vi "Wrap value.vi"(1 "Starting Angle":dbl min=0.0 max=360.0 step=1.0, 2 "Change":dbl) -> (0 "Num":dbl)   [LabVIEW 2016]
doc: "Essentially the mod function.....\n\nCreated by Team 4130 for use in the 2016-2017 FRC season"
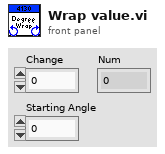
[diagram p1: front panel]
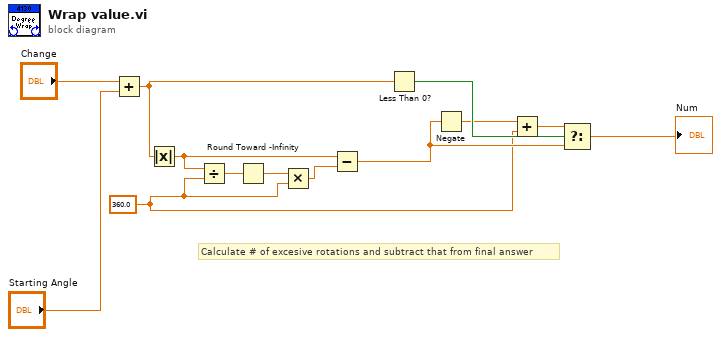
[diagram p0: block diagram]
diagram:
  w6 = 360.0
  # "Calculate # of excesive rotations and subtract that from final answer"
  n1 = Add(x="Change", y="Starting Angle") -> (x+y=w1:dbl)
  n2 = Absolute Value(x=w1) -> (abs(x)=w11:dbl)
  n3 = Divide(x=w11, y=w6) -> (x/y=w13:dbl)
  n4 = Round Toward -Infinity(1:w13) -> (0:w12:dbl)
  n5 = Multiply(x=w12, y=w6) -> (x*y=w10:dbl)
  n6 = Subtract(x=w11, y=w10) -> (x-y=w9:dbl)
  n7 = Less Than 0?(x=w1) -> (x < 0?=w8:bool)
  n8 = Negate(x=w9) -> (-x=w7:dbl)
  n9 = Add(x=w7, y=w6) -> (x+y=w5:dbl)
  n10 = Select(t=w5, s=w8, f=w9) -> (s? t:f=→"Num":dbl)
